vi "Write Disabled.vi"(8 "error in (no error)":errorcluster, 10 "Disabled":T1(ring), 11 "Disabled Assertion in":refnum<class "Disabled Assertion.lvclass">) -> (0 "error out":errorcluster, 3 "Disabled Assertion out":refnum<class "Disabled Assertion.lvclass">)   [LabVIEW 2020, in "MacroAssert.lvlib" / "Disabled Assertion.lvclass"]
uses:
  Disabled Assertion.lvclass
  Disabled Assertion.lvclass/Disabled Assertion.ctl
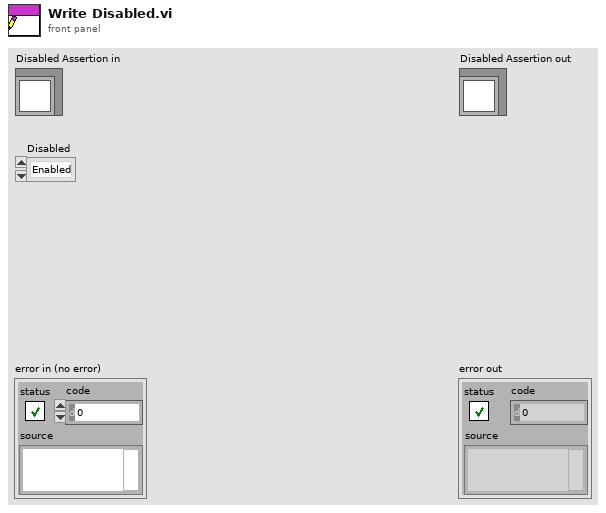
[diagram p1: front panel]
types:
  T1 = enum8{"Enabled", "Disabled", "Disabled and Grayed Out"}
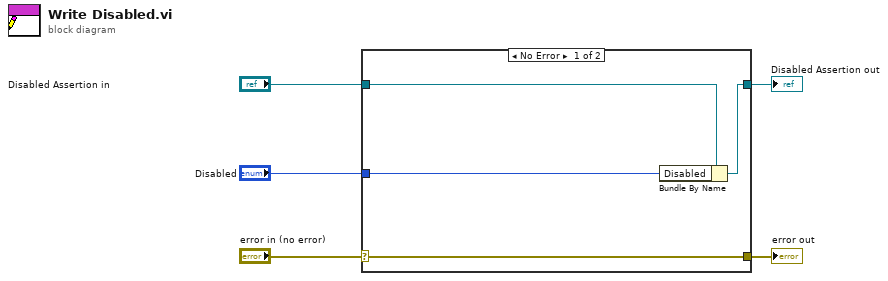
[diagram p0: block diagram]
diagram:
  n1 = case shown="No Error" "error in (no error)" {
    selector: "error in (no error)" -> [w9 w10]
    tunnel: [w9 w10] -> w4
    tunnel: [w7 w11] -> w2
    tunnel: "Disabled Assertion in" -> [w8 w11]
    tunnel: "Disabled" -> [w6 _]
    frame No Error {
      n2 = Bundle By Name(cluster=w8, "Disabled"=w6) -> (w7:refnum<class "Disabled Assertion.lvclass">)
    }
    frame Error {
    }
  }
  "error out" <- w4
  "Disabled Assertion out" <- w2
